vi "SSL Detection Ball Distance.vi"(10 "Detection Ball":T1, 11 "Detection Ball 2":T1) -> (3 "norm":dbl)   [LabVIEW 2016]
uses:
  SSL Detection Ball.ctl
  <vilib>/Analysis/_algsub.llb/Vector Norm Type.ctl
  <vilib>/Analysis/_algsub.llb/Real Vector Norm.vi
  <vilib>/Analysis/NI_AALPro.lvlib
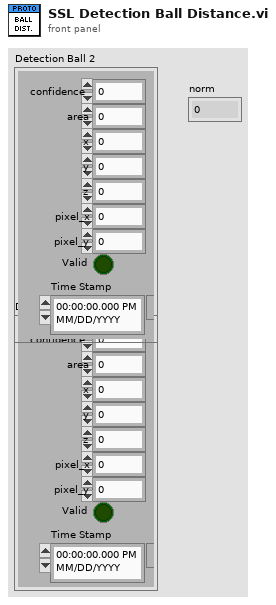
[diagram p1: front panel]
types:
  T1 = typedef "SSL Detection Ball.ctl" = cluster{"x":sgl, "area":u32, "confidence":sgl, "y":sgl, "z":sgl, "pixel_x":sgl, "pixel_y":sgl, "Valid":bool, "Time Stamp":timestamp}
  T2 = typedef "NI_AALPro.lvlib/Vector Norm Type.ctl" = u16
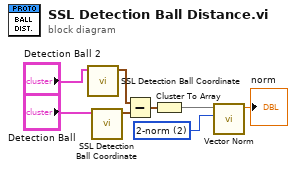
[diagram p0: block diagram]
diagram:
  w4 = T2 2 items=["1-norm"=1, "2-norm"=2, "Inf-norm"=3, "-Inf-norm"=4, "User Defined"=5] ("norm type")
  n1 = call "SSL Detection Ball Coordinate.vi"("Detection Ball"="Detection Ball 2") -> ("Coordinate"=w5:cluster{"x":sgl, "y":sgl, "z":sgl})  [unwired: 10 in]
  n2 = call "SSL Detection Ball Coordinate.vi"("Detection Ball"="Detection Ball") -> ("Coordinate"=w1:cluster{"x":sgl, "y":sgl, "z":sgl})  [unwired: 10 in]
  n3 = Subtract(x=w5, y=w1) -> (x-y=w2:cluster{"x":sgl, "y":sgl, "z":sgl})
  n4 = Cluster To Array(cluster=w2) -> (array=w3:sgl[])
  n5 = call-poly <vilib>:"Vector Norm.vi"("norm type"=w4, "Input Vector"=w3) -> ("norm"=→"norm":dbl)  [unwired: 8 in, 1 out]
